vi "harp_write_reg.vi"(0 "port":refnum<visa-resource-name>, 1 "16 bits":u16, 2 "32 bits":u32, 3 "64 bits":u64, 4 "float":sgl, 5 "error in (no error)":errorcluster, 6 "8 bits":u8 format="%x", 7 "bool":bool, 8 "8 bits (array)":u8[](array[numeric]), 9 "Array?":bool, 10 "port":u8, 11 "type":u8(ring)=1 items=["U8"=1, "U16"=2, "U32"=4, "U64"=8, "I8"=129, "I16"=130, "I32"=132, "I64"=136, "FLOAT"=68, "BOOL"=17], 12 "reg. address":u8) -> (13 "timestamp":dbl format="%.6f", 14 "port out":refnum<visa-resource-name>, 19 "error out":errorcluster)   [LabVIEW 2010]
uses:
  <vilib>/Instr/_visa.llb/VISA Flush IO Buffer Mask.ctl
panel:
  in  "32 bits 2":u32
  in  "float 2":sgl
  in  "16 bits 2":u16
  in  "64 bits 2":u64
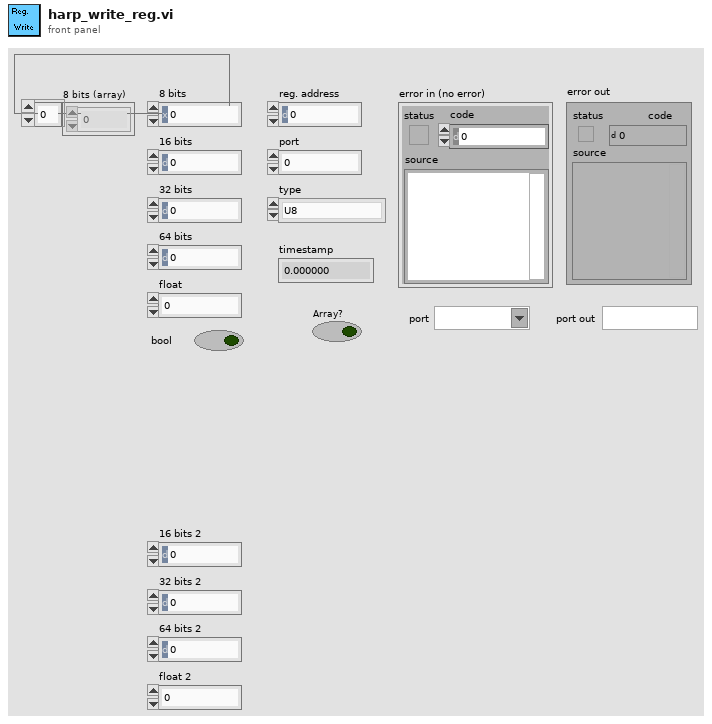
[diagram p1: front panel]
types:
  T1 = typedef "VISA Flush IO Buffer Mask.ctl" = u16
  T2 = enum16{"big-endian, network order", "native, host order", "little-endian"}
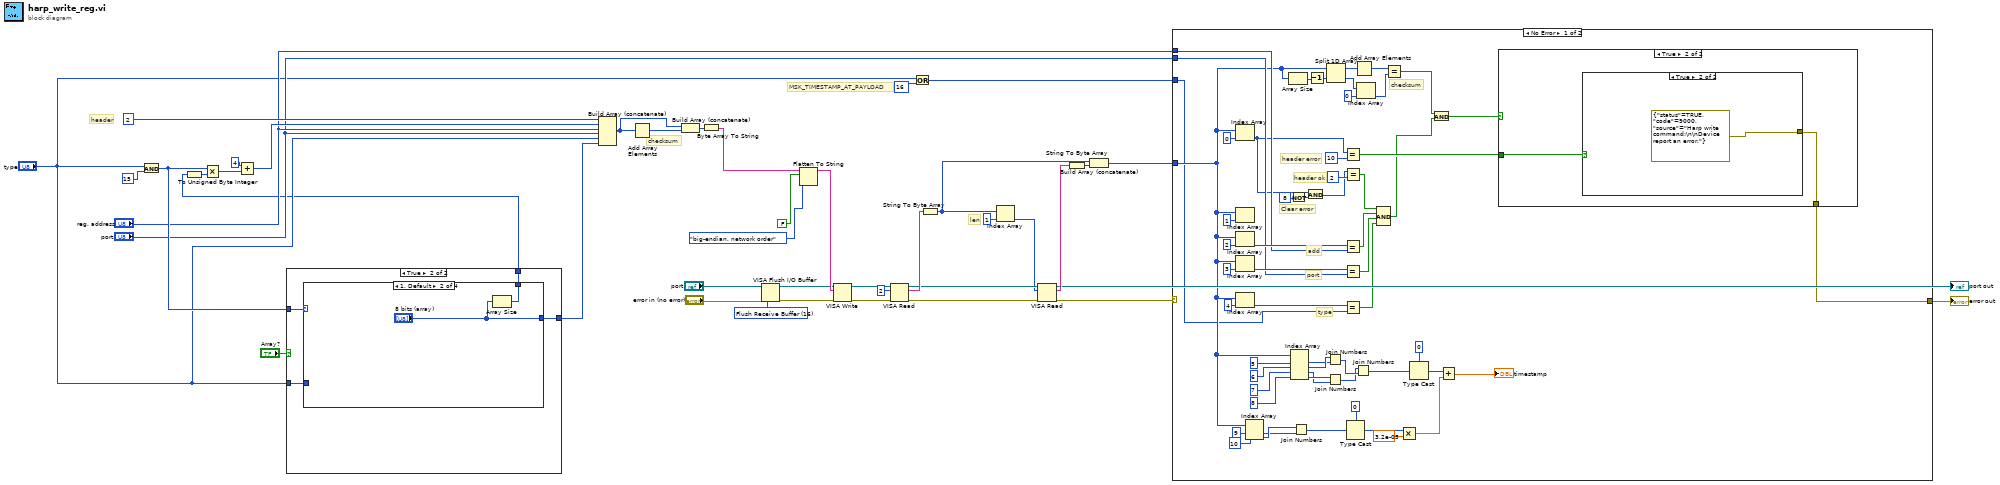
[diagram p0: block diagram]
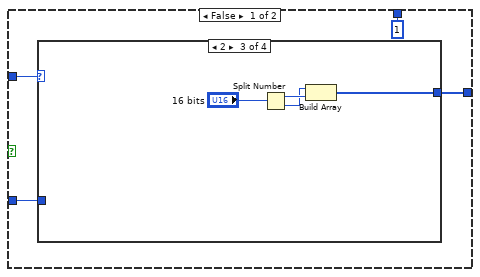
[diagram p2: hidden frame]
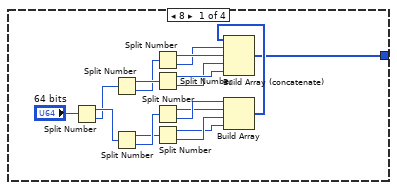
[diagram p3: hidden frame]
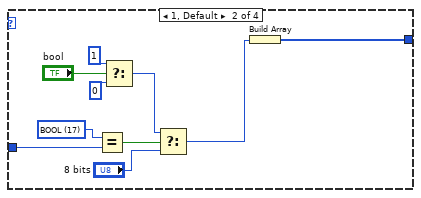
[diagram p4: hidden frame]
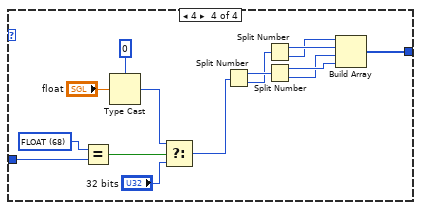
[diagram p5: hidden frame]
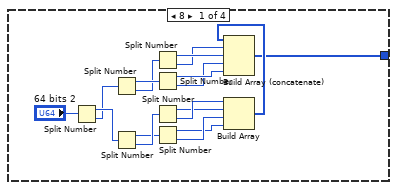
[diagram p6: hidden frame]
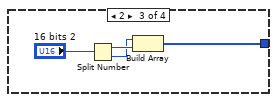
[diagram p7: hidden frame]
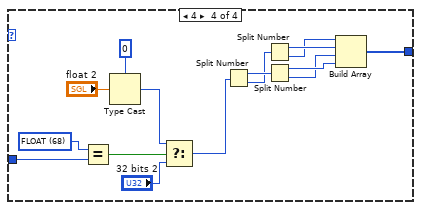
[diagram p8: hidden frame]
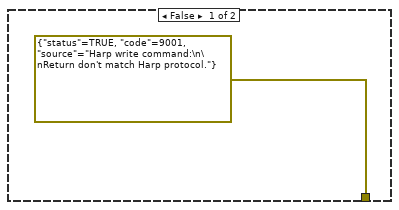
[diagram p9: hidden frame]
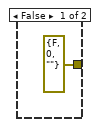
[diagram p10: hidden frame]
diagram:
  w29 = T1 16 items=["Flush Receive Buffer"=16, "Write Transmit Buffer to Device"=32, "Flush Receive Buffer (No I/O)"=64, "Flush Transmit Buffer"=128] ("Mask")
  # "MSK_TIMESTAMP_AT_PAYLOAD"
  # "len"
  # "checksum"
  # "header"
  n1 = And(x="type", y=u8 15) -> (x .and. y?=w34:u8)
  n2 = case shown="True" "Array?" {
    tunnel: w34 -> [w46 w94]
    tunnel: [w45 w96] -> w3
    tunnel: "type" -> [w44 w95]
    tunnel: [1 w93] -> w1
    frame False {
      n3 = case shown="2" w46 {
        tunnel: [w47 w73 w74 w86] -> w45
        tunnel: w44 -> [_ w71 _ w85]
        frame 8 {
          n4 = Split Number(x="64 bits") -> (hi(x)=w62:u32, lo(x)=w61:u32)
          n5 = Split Number(x=w61) -> (hi(x)=w52:u16, lo(x)=w51:u16)
          n6 = Split Number(x=w62) -> (hi(x)=w57:u16, lo(x)=w58:u16)
          n7 = Split Number(x=w51) -> (hi(x)=w50:u8, lo(x)=w49:u8)
          n8 = Split Number(x=w52) -> (hi(x)=w54:u8, lo(x)=w53:u8)
          n9 = Split Number(x=w58) -> (hi(x)=w59:u8, lo(x)=w60:u8)
          n10 = Split Number(x=w57) -> (hi(x)=w55:u8, lo(x)=w56:u8)
          n11 = Build Array(w60, w59, w56, w55) -> (w48:u8[])
          n12 = Build Array (concatenate)(w48, w49, w50, w53, w54) -> (w47:u8[])
        }
        frame 1, Default {
          w72 = u8 17 items=["U8"=1, "U16"=2, "U32"=4, "U64"=8, "I8"=129, "I16"=130, "I32"=132, "I64"=136, "FLOAT"=68, "BOOL"=17] ("type 2")
          n13 = Equal?(x=w72, y=w71) -> (x = y?=w70:bool)
          n14 = Select(t=u8 1 ("8 bits"), s="bool", f=u8 0 ("8 bits")) -> (s? t:f=w68:u8)
          n15 = Select(t=w68, s=w70, f="8 bits") -> (s? t:f=w65:u8)
          n16 = Build Array(w65) -> (w73:u8[])
        }
        frame 2 {
          n17 = Split Number(x="16 bits") -> (hi(x)=w76:u8, lo(x)=w75:u8)
          n18 = Build Array(w75, w76) -> (w74:u8[])
        }
        frame 4 {
          w84 = u8 68 items=["U8"=1, "U16"=2, "U32"=4, "U64"=8, "I8"=129, "I16"=130, "I32"=132, "I64"=136, "FLOAT"=68, "BOOL"=17] ("type 2")
          n19 = Equal?(x=w84, y=w85) -> (x = y?=w81:bool)
          n20 = Type Cast(type=u32 0 ("byte count"), x="float") -> (*(type *) &x=w80:u32)
          n21 = Select(t=w80, s=w81, f="32 bits") -> (s? t:f=w78:u32)
          n22 = Split Number(x=w78) -> (hi(x)=w90:u16, lo(x)=w89:u16)
          n23 = Split Number(x=w89) -> (hi(x)=w88:u8, lo(x)=w87:u8)
          n24 = Split Number(x=w90) -> (hi(x)=w92:u8, lo(x)=w91:u8)
          n25 = Build Array(w87, w88, w91, w92) -> (w86:u8[])
        }
      }
    }
    frame True {
      n26 = case shown="1, Default" w94 {
        tunnel: [w97 "8 bits (array)" w116 w128] -> w96
        tunnel: w95 -> [_ _ _ w127]
        tunnel: [_ w114 _ _] -> w93
        frame 8 {
          n27 = Split Number(x="64 bits 2") -> (hi(x)=w112:u32, lo(x)=w111:u32)
          n28 = Split Number(x=w111) -> (hi(x)=w102:u16, lo(x)=w101:u16)
          n29 = Split Number(x=w112) -> (hi(x)=w107:u16, lo(x)=w108:u16)
          n30 = Split Number(x=w101) -> (hi(x)=w100:u8, lo(x)=w99:u8)
          n31 = Split Number(x=w102) -> (hi(x)=w104:u8, lo(x)=w103:u8)
          n32 = Split Number(x=w108) -> (hi(x)=w109:u8, lo(x)=w110:u8)
          n33 = Split Number(x=w107) -> (hi(x)=w105:u8, lo(x)=w106:u8)
          n34 = Build Array(w110, w109, w106, w105) -> (w98:u8[])
          n35 = Build Array (concatenate)(w98, w99, w100, w103, w104) -> (w97:u8[])
        }
        frame 1, Default {
          n36 = Array Size(array="8 bits (array)") -> (size(s)=w114:i32)
        }
        frame 2 {
          n37 = Split Number(x="16 bits 2") -> (hi(x)=w118:u8, lo(x)=w117:u8)
          n38 = Build Array(w117, w118) -> (w116:u8[])
        }
        frame 4 {
          w126 = u8 68 items=["U8"=1, "U16"=2, "U32"=4, "U64"=8, "I8"=129, "I16"=130, "I32"=132, "I64"=136, "FLOAT"=68, "BOOL"=17] ("type 2")
          n39 = Equal?(x=w126, y=w127) -> (x = y?=w123:bool)
          n40 = Type Cast(type=u32 0 ("byte count"), x="float 2") -> (*(type *) &x=w122:u32)
          n41 = Select(t=w122, s=w123, f="32 bits 2") -> (s? t:f=w120:u32)
          n42 = Split Number(x=w120) -> (hi(x)=w132:u16, lo(x)=w131:u16)
          n43 = Split Number(x=w131) -> (hi(x)=w130:u8, lo(x)=w129:u8)
          n44 = Split Number(x=w132) -> (hi(x)=w134:u8, lo(x)=w133:u8)
          n45 = Build Array(w129, w130, w133, w134) -> (w128:u8[])
        }
      }
    }
  }
  n46 = To Unsigned Byte Integer(number=w1) -> (unsigned 8bit integer=w2:u8)
  n47 = Multiply(x=w34, y=w2) -> (x*y=w4:u8)
  n48 = Add(x=u8 4, y=w4) -> (x+y=w36:u8)
  n49 = Build Array (concatenate)(u8 2 ("element"), w36, "reg. address", "port", "type", w3) -> (w24:u8[])
  n50 = Add Array Elements(numeric array=w24) -> (sum=w25:u8)
  n51 = Build Array (concatenate)(w24, w25) -> (w23:u8[])
  n52 = Byte Array To String(unsigned byte array=w23) -> (string=w38:string)
  n53 = VISA Flush I/O Buffer(VISA resource name="port", mask (16)=w29, error in (no error)="error in (no error)") -> (VISA resource name out=w32:refnum<visa-resource-name>, error out=w33:errorcluster)
  n54 = Flatten To String(anything=w38, prepend array or string size? (T)=FALSE, byte order (0:big-endian, network order)=T2."big-endian, network order") -> (data string=w40:string)  [unwired: 1 in, 2 out]
  n55 = VISA Write(VISA resource name=w32, write buffer=w40, error in (no error)=w33) -> (VISA resource name out=w12:refnum<visa-resource-name>, error out=w13:errorcluster)  [unwired: 1 out]
  n56 = VISA Read(VISA resource name=w12, byte count=u32 2, error in (no error)=w13) -> (VISA resource name out=w19:refnum<visa-resource-name>, read buffer=w20:string, error out=w18:errorcluster)  [unwired: 1 out]
  n57 = Or(x="type", y=u8 16) -> (x .or. y?=w6:u8)
  n58 = String To Byte Array(string=w20) -> (unsigned byte array=w14:u8[])
  n59 = Index Array(array=w14, index=1) -> (element=w15:u8)
  n60 = VISA Read(VISA resource name=w19, byte count=w15, error in (no error)=w18) -> (VISA resource name out=→"port out":refnum<visa-resource-name>, read buffer=w17:string, error out=w10:errorcluster)  [unwired: 1 out]
  n61 = String To Byte Array(string=w17) -> (unsigned byte array=w16:u8[])
  n62 = Build Array (concatenate)(w14, w16) -> (w11:u8[])
  n63 = case shown="No Error" w10 {
    selector: w10 -> [_ w197]
    tunnel: [w186 w197] -> w28
    tunnel: "reg. address" -> [w185 _]
    tunnel: "port" -> [w182 _]
    tunnel: w11 -> [w142 _]
    tunnel: w6 -> [w141 _]
    frame No Error {
      # "Clear error"
      # "type"
      # "checksum"
      # "header error"
      # "port"
      # "add"
      # "header ok"
      n64 = Index Array(array=w142, index=0) -> (element=w136:u8)
      n65 = Index Array(array=w142, index=1) -> ()  [unwired: 1 out]
      n66 = Index Array(array=w142, index=2) -> (element=w188:u8)
      n67 = Index Array(array=w142, index=3) -> (element=w183:u8)
      n68 = Index Array(array=w142, index=4) -> (element=w143:u8)
      n69 = Index Array(array=w142, index #1=9 ("index"), index #2=10 ("index")) -> (element #1=w150:u8, element #2=w151:u8)
      n70 = Array Size(array=w142) -> (size(s)=w178:i32)
      n71 = Not(x=u8 8 ("y")) -> (.not. x?=w138:u8)
      n72 = Index Array(array=w142, index #1=5 ("index"), index #2=6 ("index"), index #3=7 ("index"), index #4=8 ("index")) -> (element #1=w161:u8, element #2=w165:u8, element #3=w162:u8, element #4=w163:u8)
      n73 = Join Numbers(hi=w151, lo=w150) -> ((hi.lo)=w152:u16)
      n74 = And(x=w136, y=w138) -> (x .and. y?=w137:u8)
      n75 = Decrement(x=w178) -> (x-1=w177:i32)
      n76 = Join Numbers(hi=w165, lo=w161) -> ((hi.lo)=w166:u16)
      n77 = Join Numbers(hi=w163, lo=w162) -> ((hi.lo)=w164:u16)
      n78 = Split 1D Array(array=w142, index=w177) -> (first subarray=w176:u8[], second subarray=w173:u8[])
      n79 = Equal?(x=w136, y=u8 10) -> (x = y?=w180:bool)
      n80 = Equal?(x=w188, y=w185) -> (x = y?=w146:bool)
      n81 = Equal?(x=w183, y=w182) -> (x = y?=w145:bool)
      n82 = Equal?(x=w143, y=w141) -> (x = y?=w140:bool)
      n83 = Equal?(x=w137, y=u8 2) -> (x = y?=w135:bool)
      n84 = Type Cast(type=u16 0 ("byte count"), x=w152) -> (*(type *) &x=w154:u16)
      n85 = Join Numbers(hi=w164, lo=w166) -> ((hi.lo)=w156:u32)
      n86 = Add Array Elements(numeric array=w176) -> (sum=w175:u8)
      n87 = Index Array(array=w173, index=0) -> (element=w172:u8)
      n88 = Compound Arithmetic op=AND(w135, w146, w145, w140) -> (w170:bool)
      n89 = Equal?(x=w175, y=w172) -> (x = y?=w171:bool)
      n90 = Multiply(x=w154, y=3.2e-05) -> (x*y=w169:dbl)
      n91 = Type Cast(type=u32 0 ("byte count"), x=w156) -> (*(type *) &x=w168:u32)
      n92 = And(x=w171, y=w170) -> (x .and. y?=w179:bool)
      n93 = Add(x=w168, y=w169) -> (x+y=→"timestamp":dbl)
      n94 = case shown="True" w179 {
        tunnel: [errorcluster {"status"=TRUE, "code"=9001, "source"="Harp write command:\n\nReturn don't match Harp protocol."} ("error out") w194] -> w186
        tunnel: w180 -> [_ w193]
        frame False {
        }
        frame True {
          n95 = case shown="True" w193 {
            tunnel: [errorcluster {"status"=FALSE, "code"=0, "source"=""} ("error out") errorcluster {"status"=TRUE, "code"=9000, "source"="Harp write command:\n\nDevice report an error."} ("error out")] -> w194
            frame False {
            }
            frame True {
            }
          }
        }
      }
    }
    frame Error {
    }
  }
  "error out" <- w28
